vi "Exemple_Metrics_Fbeta_Score.vi"() -> ()   [LabVIEW 2020]
uses:
  Objet/3 - Model selection and evaluation/3.3 - Metrics and scoring/fbeta_score/Fbeta_Score.vi
panel:
  out "Data":T1
  out "error out":errorcluster caption="sortie d'erreur"
  in  "fbeta_score":T2={"beta"=0.5, "labels"=[], "pos_label"={"dtype_pos_label"="int", "pos_label"="1"}, "average"="None", "sample_weight"=[], "zero_division"={"dtype_zero_division"="str", "zero_division"="warn"}}
  in  "error in (no error)":errorcluster caption="entrée d'erreur (pas d'erreur)"
  in  "y_pred":string[][](array[string])=[["0"], ["2"], ["1"], ["0"], ["0"], ["1"]]
  in  "y_true":string[][](array[string])=[["0"], ["1"], ["2"], ["0"], ["1"], ["2"]]
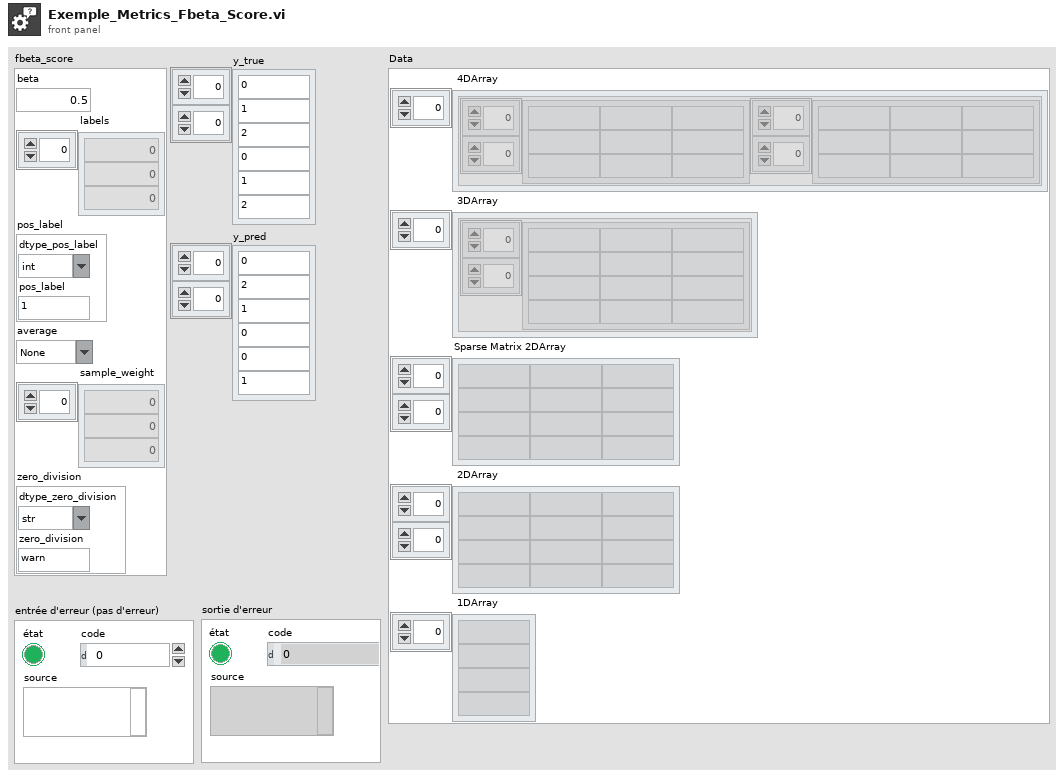
[diagram p1: front panel]
types:
  T1 = cluster{" 4DArray":cluster{"1":string[][], "2":string[][]}[], " 3DArray":cluster{"Tableau":string[][]}[], "Sparse Matrix 2DArray":string[][], " 2DArray":string[][], " 1DArray":string[]}
  T2 = cluster{"beta":dbl, "labels":i32[], "pos_label":cluster{"dtype_pos_label":string, "pos_label":string}, "average":string, "sample_weight":dbl[], "zero_division":cluster{"dtype_zero_division":string, "zero_division":string}}
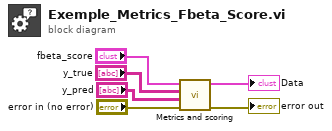
[diagram p0: block diagram]
diagram:
  n1 = call-poly "Metrics and scoring.vi"("error in (no error)"="error in (no error)", "y_pred"="y_pred", "y_true"="y_true", "fbeta_score"="fbeta_score") -> ("error out"=→"error out":errorcluster, "Data"=→"Data":T1)  [unwired: 6 in]
